vi "dfd_Filter Signal by Coef.vi"(6 "state in":dbl[](array[numeric]), 7 "initH?":bool, 8 "error in(no error)":errorcluster, 9 "coef source":enum16{"Original", "Current", "Quantized"}(ring)=enum."Current", 10 "filter":T1={"mSRate_Fs"=1.0, "mSRate_Version"="1.0", "mSRate_Comments"="", "mSRate_OrgCoef"={"type"=enum."Undefined", "gain"=1.0, "coef a (k)"=[], "coef b (v)"=[]}, "mSRate_CurCoef"={"type"=enum."Undefined", "gain"=1.0, "coef a (k)"=[], "coef b (v)"=[]}, "mSRate_Quantized?"=FALSE, "mSRate_QCoef"={"type"=enum."Undefined", "gain"=1.0, "coef a (k)"=[], "coef b (v)"=[]}, "mSRate_QSettings"=[], "mSRate_Order"=0, "mSRate_Scaling"={"mSRate_ScaleByPowerOf2?"=FALSE, "mSRate_ScaleType"=enum."No Norm"}} {"mSRate_QSettings"."source" items=["Coef a/k"=0, "Coef b/v"=7, "Input"=1, "Output"=2, "Multiplicand"=3, "Product"=4, "Sum"=5, "Delay"=6, "Gain"=8]}, 11 "x":dbl[](array[numeric])) -> (0 "error out":errorcluster, 3 "filtered x":dbl[](array[numeric]), 4 "state out":dbl[](array[numeric]))   [LabVIEW 2017, in "NI_DigFilterLicensed.lvlib"]
uses:
  <vilib>/addons/Digital Filter Design/NI_DigFilterLicensed.lvlib
  <vilib>/addons/Digital Filter Design/_Objects.llb/DFD Filter Obj.ctl
  <vilib>/addons/Digital Filter Design/_Objects.llb/DFD Filter Coef.ctl
  <vilib>/addons/Digital Filter Design/_Objects.llb/DFD Filter Structure Type Selector.ctl
  <vilib>/addons/Digital Filter Design/_Objects.llb/dfd_Internal Quantization Settings.ctl
  <vilib>/addons/Digital Filter Design/_Objects.llb/dfd_Internal Quantization Srcs.ctl
  <vilib>/addons/Digital Filter Design/_Objects.llb/DFD Coef Norm Type.ctl
  <resource>/LVDFD.dll
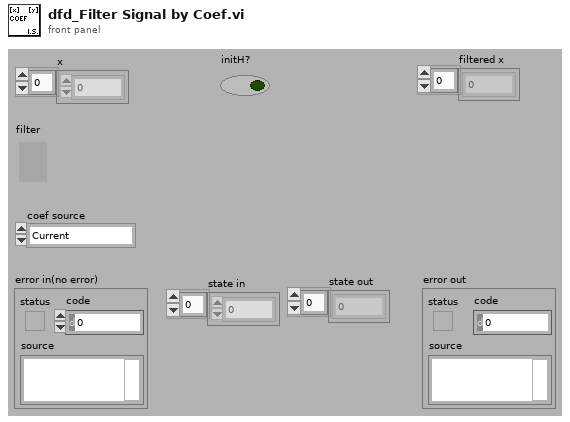
[diagram p1: front panel]
types:
  T1 = typedef "NI_DigFilterLicensed.lvlib/DFD Filter Obj.ctl" = cluster{"mSRate_Fs":dbl, "mSRate_Version":string, "mSRate_Comments":string, "mSRate_OrgCoef":T2, "mSRate_CurCoef":T2, "mSRate_Quantized?":bool, "mSRate_QCoef":T2, "mSRate_QSettings":T4[], "mSRate_Order":i32, "mSRate_Scaling":cluster{"mSRate_ScaleByPowerOf2?":bool, "mSRate_ScaleType":T6}}
  T2 = typedef "NI_DigFilterLicensed.lvlib/DFD Filter Coef.ctl" = cluster{"type":T3, "gain":dbl, "coef a (k)":dbl[], "coef b (v)":dbl[]}
  T3 = typedef "NI_DigFilterLicensed.lvlib/DFD Filter Structure Type Selector.ctl" = enum16{"Undefined", "FIR Direct Form", "FIR Direct Form Transposed", "FIR Symmetric", "FIR Antisymmetric", "IIR Direct Form I", "IIR Direct Form I Transposed", "IIR Direct Form II", "IIR Direct Form II Transposed", "IIR Cascaded Second Order Sections Form I", "IIR Cascaded Second Order Sections Form I Transposed", "IIR Cascaded Second Order Sections Form II", "IIR Cascaded Second Order Sections Form II Transposed", "Lattice Allpass (basic sections)", "Lattice Allpass (one multiplier sections)", "Lattice Allpass (normalized sections)", "Lattice AR (basic sections)", "Lattice AR (one multiplier sections)", "Lattice AR (normalized sections)", "Lattice MA (minimum phase)", "Lattice MA (maximum phase)", "Lattice ARMA (basic sections)", "Lattice ARMA (one multiplier sections)", "Lattice ARMA (normalized sections)"}
  T4 = typedef "NI_DigFilterLicensed.lvlib/dfd_Internal Quantization Settings.ctl" = cluster{"source":T5, "wl":i16, "iwl":i16, "overflow mode":enum16{"Saturation", "Wrap"}, "rounding mode":enum16{"Nearest", "Truncation"}, "signed?":bool}
  T5 = typedef "NI_DigFilterLicensed.lvlib/dfd_Internal Quantization Srcs.ctl" = u16
  T6 = typedef "NI_DigFilterLicensed.lvlib/DFD Coef Norm Type.ctl" = enum16{"No Norm", "Time Domain 1-Norm", "Time Domain 2-Norm", "Time Domain Inf-Norm"}
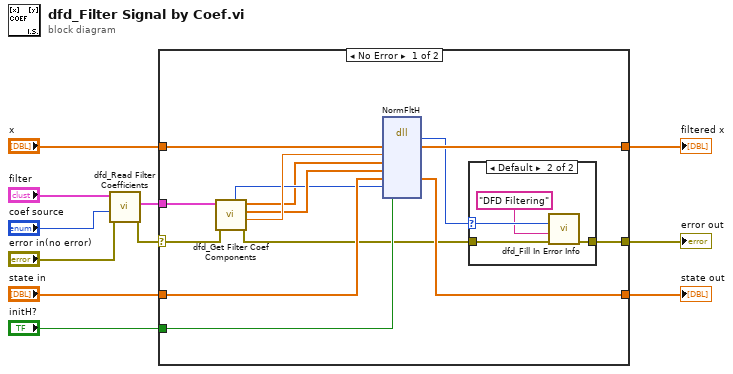
[diagram p0: block diagram]
diagram:
  n1 = call <vilib>:"dfd_Read Filter Coefficients.vi"("error in (no error)"="error in(no error)", "coef source"="coef source", "filter in"="filter") -> ("error out"=w2:errorcluster, "filter coef"=w4:T2)  [unwired: 7 out]
  n2 = case shown="No Error" w2 {
    selector: w2 -> [w12 w31]
    tunnel: "state in" -> [w22 _]
    tunnel: [w21 _] -> w10
    tunnel: [w18 w31] -> w9
    tunnel: "x" -> [w25 _]
    tunnel: [w20 _] -> w7
    tunnel: "initH?" -> [w17 _]
    tunnel: w4 -> [w13 _]
    frame No Error {
      n3 = call <vilib>:"dfd_Get Filter Coef Components.vi"("error in (no error)"=w12, "filter coef"=w13) -> ("error out"=w16:errorcluster, "gain"=w24:dbl, "coef a (k)"=w23:dbl[], "coef b (v)"=w14:dbl[], "type"=w15:T3)  [unwired: 5 out]
      n4 = dll-call lib="C:/Program Files/National Instruments/LabVIEW 2017/resource/LVDFD.dll" fn="NormFltH" ("Call Library Node")("inputDataH"=w25, "gainH"=w24, "coefBH"=w14, "coefAH"=w23, "statesH"=w22, "type"=w15, "initH"=w17) -> ("return value"=w19:i32, "inputDataH"=w20:dbl[], "statesH"=w21:dbl[])  [unwired: 7 in, 3 out]
      n5 = case shown="Default" w19 {
        selector: w19 -> [_ w28]
        tunnel: w16 -> [w26 w30]
        tunnel: [w26 w29] -> w18
        frame 0 {
        }
        frame Default {
          n6 = call <vilib>:"dfd_Fill In Error Info.vi"("error in"=w30, "extended error info"="DFD Filtering", "status code"=w28) -> ("error out"=w29:errorcluster)  [unwired: 1 in, 7 out]
        }
      }
    }
    frame Error {
    }
  }
  "state out" <- w10
  "error out" <- w9
  "filtered x" <- w7
